vi "ProcessErrorHandle.vi"(8 "error in (no error)":errorcluster) -> (0 "error out (no error)":errorcluster)   [LabVIEW 2019]
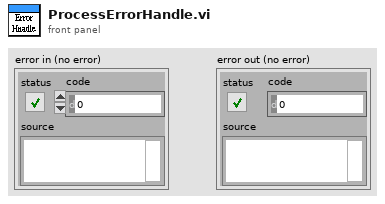
[diagram p1: front panel]
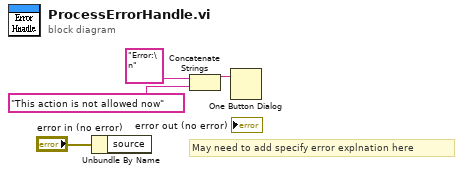
[diagram p0: block diagram]
diagram:
  # "May need to add specify error explnation here"
  n1 = Unbundle By Name("error in (no error)") -> ()  [unwired: 1 out]
  n2 = Concatenate Strings("Error:\n" ("string"), "This action is not allowed now" ("string")) -> (w4:string)
  n3 = One Button Dialog(message=w4) -> ()  [unwired: 1 in, 1 out]
